vi "Conv1D.vi"() -> ()   [LabVIEW 2020]
doc: "This benchmark is designed to demonstrate execution performance improvement when executing FFT and IFFT operations on a GPU."
uses:
  956bade7-a26b-4376-82d1-4f43b9b25d0c.vi
  a45b64e6-426e-4566-b00d-58499d731ec9.vi
  2d4acfdf-3b2f-4360-8aac-546d4cc334b7.vi
  e3d6266a-341e-462f-8124-2d714a455819.vi
  <vilib>/Analysis/2dsp.llb/1D Convolution (DBL).vi
  <vilib>/Utility/High Resolution Relative Seconds.vi
  <vilib>/Ngene/CuLab - GPU Accelerated Toolkit/Toolkit/Low_Level/Tensor_Classes/T_Children/T1D/T1D_Children/T1D_SGL/Pull.vi
  <vilib>/Ngene/CuLab - GPU Accelerated Toolkit/Toolkit/API/Signal Processing/Signal Operation/Convolution/T1D/CU_Convolution_T1D_SGL.vi
  <vilib>/Ngene/CuLab - GPU Accelerated Toolkit/Toolkit/Low_Level/Tensor_Classes/T_Children/T1D/T1D_Children/T1D_SGL/Push.vi
  <vilib>/Ngene/CuLab - GPU Accelerated Toolkit/Toolkit/Low_Level/Tensor_Classes/T_Children/T1D/T1D_Children/T1D_SGL/Create_Push.vi
  <vilib>/Analysis/NI_AALBase.lvlib
  <vilib>/Ngene/CuLab - GPU Accelerated Toolkit/Toolkit/CuLab.lvlib
  <vilib>/Analysis/NI_AALPro.lvlib
  <vilib>/Ngene/CuLab - GPU Accelerated Toolkit/Toolkit/Low_Level/Tensor_Classes/T_Children/T1D/T1D_Children/T1D_SGL/T1D_SGL.lvclass
panel:
  out "CPU (sec)":dbl[](array[numeric])=[42.131092355985324, 35.429105230316075, 31.16246342351057, 25.767502048252396, 19.87054670676759, 14.576277208271852, 12.74999997084953, 7.518399561317554, 3.7424450318208833, 2.0503842820924176, 0.9362123659453822, 0.46770236324055325, 0.27725117698960117, 0.09920318843476397, 0.09302326738770976, 0.05329593103290103, 0.030920595781795512] format="%_3p"
  out "GPU (sec)":dbl[](array[numeric])=[42.131092355985324, 35.429105230316075, 31.16246342351057, 25.767502048252396, 19.87054670676759, 14.576277208271852, 12.74999997084953, 7.518399561317554, 3.7424450318208833, 2.0503842820924176, 0.9362123659453822, 0.46770236324055325, 0.27725117698960117, 0.09920318843476397, 0.09302326738770976, 0.05329593103290103, 0.030920595781795512] format="%_3p"
  out "Kernel Sizes":i32[](array[numeric])=[8389, 4195, 2098, 1049, 525, 263, 132, 66, 33, 17, 9, 5, 3, 3, 3, 3, 3] format="%#.7f"
  out "SpeedUp":dbl[](array[numeric])=[42.131092355985324, 35.429105230316075, 31.16246342351057, 25.767502048252396, 19.87054670676759, 14.576277208271852, 12.74999997084953, 7.518399561317554, 3.7424450318208833, 2.0503842820924176, 0.9362123659453822, 0.46770236324055325, 0.27725117698960117, 0.09920318843476397, 0.09302326738770976, 0.05329593103290103, 0.030920595781795512] format="%.2f"
  in  "Kernel Relative Size":sgl=0.001
  out "Iteration":i32=9
  out "FFT_Size":i32=128
  out "Status":string="Computing on CPU"
  out "GPU Model":string="NVIDIA GeForce GTX 1650 Ti"
  out "CPU Model":string="Intel(R) Core(TM) i7-10750H CPU @ 2.60GHz  "
  in  "No. of Repetitions":i32=10
  in  "Signal Size Stop (2^N)":i32=23
  in  "Signal Size Start (2^N)":i32=7
  out "Signal Sizes":i32[](array[numeric])=[8388608, 4194304, 2097152, 1048576, 524288, 262144, 131072, 65536, 32768, 16384, 8192, 4096, 2048, 1024, 512, 256, 128] format="%#.4f"
  out "Performance Improvement":cluster{i32[], dbl[]}(graph)={[8388608, 4194304, 2097152, 1048576, 524288, 262144, 131072, 65536, 32768, 16384, 8192, 4096, 2048, 1024, 512, 256, 128], [42.131092355985324, 35.429105230316075, 31.16246342351057, 25.767502048252396, 19.87054670676759, 14.576277208271852, 12.74999997084953, 7.518399561317554, 3.7424450318208833, 2.0503842820924176, 0.9362123659453822, 0.46770236324055325, 0.27725117698960117, 0.09920318843476397, 0.09302326738770976, 0.05329593103290103, 0.030920595781795512]}
  out "Execution Times":cluster{i32[], "FFT mean Exec Time":dbl[]}[](graph)=[{[8388608, 4194304, 2097152, 1048576, 524288, 262144, 131072, 65536, 32768, 16384, 8192, 4096, 2048, 1024, 512, 256, 128], "FFT mean Exec Time"=[0.8448884999997972, 0.3735822000016924, 0.16075780000028317, 0.06971139999950537, 0.02983959999983199, 0.012325700001383666, 0.005569199998717522, 0.00257430000056047, 0.0010898000000452157, 0.0004802000003110152, 0.00023630000214325264, 0.00011439999798312783, 5.8499997976468876e-05, 2.4900000425986946e-05, 1.3600001693703234e-05, 7.599999662488699e-06, 4.400000761961564e-06]}, {[8388608, 4194304, 2097152, 1048576, 524288, 262144, 131072, 65536, 32768, 16384, 8192, 4096, 2048, 1024, 512, 256, 128], "FFT mean Exec Time"=[0.020053800002642674, 0.01054449999719509, 0.005158699997991789, 0.002705399998376379, 0.0015017000005173031, 0.0008455999995931052, 0.00043680000089807436, 0.0003423999987717252, 0.00029120000181137584, 0.0002342000007047318, 0.00025240000104531646, 0.0002445999998599291, 0.00021099999867146835, 0.00025100000129896216, 0.00014620000001741573, 0.00014259999807109125, 0.00014229999942472205]}]
  # "Overview: Benchmarks performance of a GPU vs CPU in 1D Convolution task.\nRequirements: PC with Nvidia GPU, with latest version of GPU driver and CuLab Toolkit installed.\nInstructions:\n1. Run the VI with the current benchmarking parameters.\n2. Wait for the completion of the execution. \nNote: It might take some time to perform the computations.\n3. Observe the timing and speedup results on the graphs."
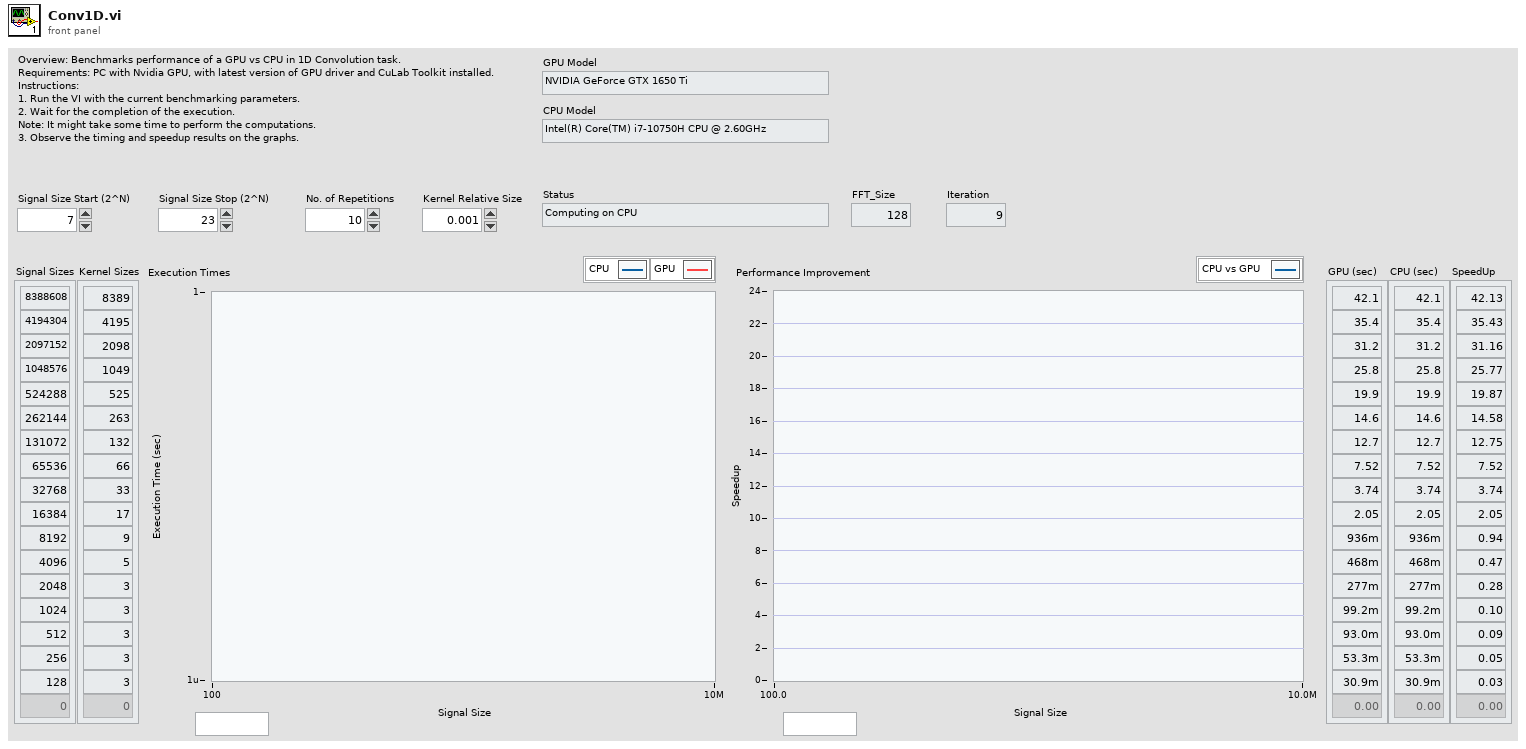
[diagram p1: front panel]
types:
  T1 = typedef "CuLab.lvlib/Properties.ctl" = cluster{"Index":i32, "Name":string}
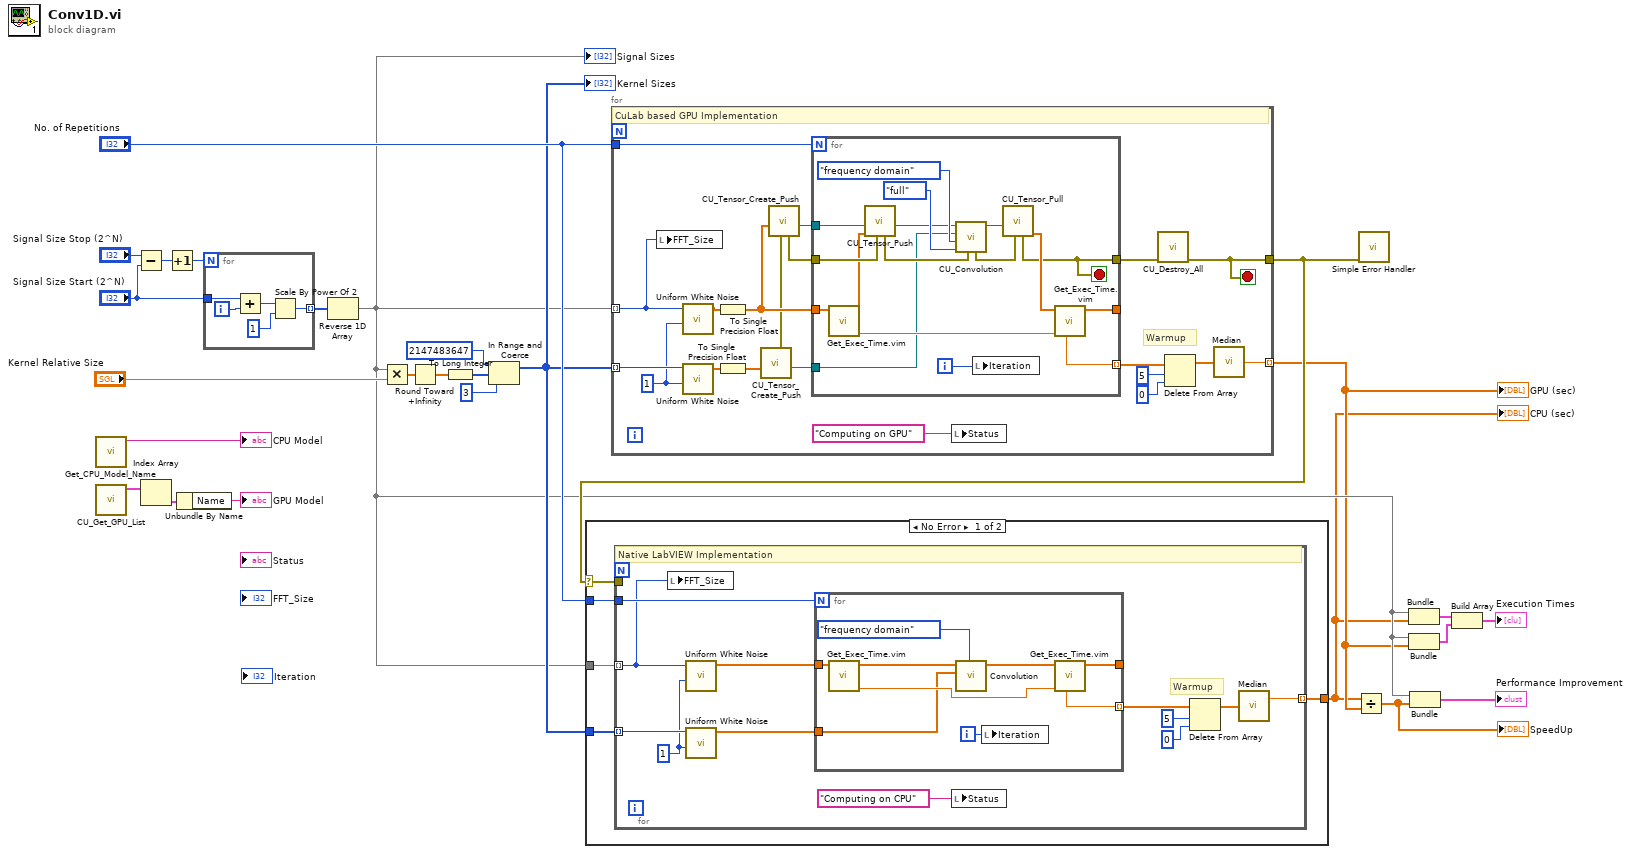
[diagram p0: block diagram]
diagram:
  n1 = call "Get_CPU_Model_Name.vi"() -> ("CPU Model"=→"CPU Model":string)  [unwired: 11 in]
  n2 = call <vilib>:"CU_Get_GPU_List.vi"() -> ("Devices"=w6:T1[])  [unwired: 10 in, 1 out]
  n3 = Subtract(x="Signal Size Stop (2^N)", y="Signal Size Start (2^N)") -> (x-y=w21:i32)
  n4 = Index Array(array=w6) -> (element=w5:T1)  [unwired: 1 in]
  n5 = Increment(x=w21) -> (x+1=w20:i32)
  n6 = Unbundle By Name(w5) -> ("Name"=→"GPU Model":string)
  n7 = for {
    N: w20 -> [_]
    tunnel: "Signal Size Start (2^N)" -> [w31]
    tunnel: [w27] -> w8 mode=indexing
    i -> [w30]
    n8 = Add(x=w31, y=w30) -> (x+y=w29:i32)
    n9 = Scale By Power Of 2(n=w29, x=1) -> (x*2^n=w27:i32)
  }
  n10 = Reverse 1D Array(array=w8) -> (reversed array=w3:i32[])
  "Signal Sizes" <- w3
  n11 = Multiply(x=w3, y="Kernel Relative Size") -> (x*y=w14:sgl[])
  n12 = Round Toward +Infinity(x=w14) -> (ceil(x): smallest int >= x=w13:sgl[])
  n13 = To Long Integer(number=w13) -> (32bit integer=w11:i32[])
  n14 = In Range and Coerce(upper limit=2147483647 ("lower limit"), x=w11, lower limit=3) -> (coerced(x)=w12:i32[])  [unwired: 1 out]
  "Kernel Sizes" <- w12
  n15 = for {
    tunnel: [w41] -> w17
    tunnel: [w49] -> w2 mode=indexing
    tunnel: w3 -> [w39] mode=indexing
    tunnel: "No. of Repetitions" -> [w45]
    tunnel: w12 -> [w33] mode=indexing
    stop <- w41 stop-if-true
    w32 = 1 ("seed")
    # "Warmup"
    # "CuLab based GPU Implementation"
    n16 = local write "FFT_Size"(w39) -> ()
    n17 = call <vilib>:"Uniform White Noise.vi"("seed"=w32, "samples"=w39) -> ("uniform white noise"=w42:dbl[])  [unwired: 8 in, 1 out]
    n18 = call <vilib>:"Uniform White Noise.vi"("seed"=w32, "samples"=w33) -> ("uniform white noise"=w38:dbl[])  [unwired: 8 in, 1 out]
    n19 = To Single Precision Float(number=w42) -> (single precision float=w43:sgl[])
    n20 = To Single Precision Float(number=w38) -> (single precision float=w37:sgl[])
    n21 = call-poly <vilib>:"CU_Tensor_Create_Push.vi"("CPU_Data_1D_SGL"=w37) -> ("T1D_SGL out"=w36:refnum<class "T1D_SGL.lvclass">, "error out"=w35:errorcluster)  [unwired: 9 in]
    n22 = call-poly <vilib>:"CU_Tensor_Create_Push.vi"("error in (no error)"=w35, "CPU_Data_1D_SGL"=w43) -> ("T1D_SGL out"=w51:refnum<class "T1D_SGL.lvclass">, "error out"=w50:errorcluster)  [unwired: 8 in]
    n23 = for {
      N: w45 -> [_]
      tunnel: w51 -> [w65]
      tunnel: w50 -> [w57]
      tunnel: [w52] -> w44
      tunnel: [w66] -> w34 mode=indexing
      tunnel: w43 -> [w56]
      tunnel: w36 -> [w58]
      tunnel: [w54] -> _
      i -> [w62]
      stop <- w52 stop-if-true
      n24 = call "Get_Exec_Time.vim"("error in (no error)"=w56) -> ("T(n)"=w67:dbl, "error out"=w55:sgl[])  [unwired: 6 in, 1 out]
      n25 = call-poly <vilib>:"CU_Tensor_Push.vi"("error in (no error)"=w57, "CPU_Data_1D_SGL"=w55, "T1D_SGL in"=w65) -> ("T1D_SGL out"=w59:refnum<class "T1D_SGL.lvclass">, "error out"=w68:errorcluster)  [unwired: 7 in]
      n26 = call-poly <vilib>:"CU_Convolution.vi"("error in"=w68, "output size"=enum32{"full", "size X", "compact"}."full", "algorithm"=enum32{"direct", "frequency domain"}."frequency domain", "Y"=w58, "X"=w59) -> ("X * Y"=w64:refnum<class "T1D_SGL.lvclass">, "error out"=w63:errorcluster)  [unwired: 5 in]
      n27 = local write "Iteration"(w62) -> ()
      n28 = call-poly <vilib>:"CU_Tensor_Pull.vi"("error in (no error)"=w63, "T1D_SGL in"=w64) -> ("Dest out"=w53:sgl[], "error out"=w52:errorcluster)  [unwired: 7 in, 1 out]
      n29 = call "Get_Exec_Time.vim"("T(n-1)"=w67, "error in (no error)"=w53) -> ("error out"=w54:sgl[], "dT"=w66:dbl)  [unwired: 5 in, 1 out]
    }
    n30 = local write "Status"("Computing on GPU" ("Info")) -> ()
    n31 = call <vilib>:"CU_Destroy_All.vi"("error in"=w44) -> ("error out"=w41:errorcluster)  [unwired: 10 in]
    n32 = Delete From Array(array=w34, length=5, index=0) -> (array with subset deleted=w48:dbl[])  [unwired: 1 out]
    n33 = call <vilib>:"Median.vi"("X"=w48) -> ("median"=w49:dbl)  [unwired: 1 out]
  }
  "GPU (sec)" <- w2
  n34 = case shown="No Error" w17 {
    selector: w17 -> [w70 _]
    tunnel: [w73 _] -> w1
    tunnel: "No. of Repetitions" -> [w72 _]
    tunnel: w3 -> [w71 _]
    tunnel: w12 -> [w69 _]
    frame No Error {
      n35 = for {
        tunnel: [w81] -> w73 mode=indexing
        tunnel: w71 -> [w77] mode=indexing
        tunnel: w72 -> [w80]
        tunnel: w70 -> [_]
        tunnel: w69 -> [w76] mode=indexing
        w74 = 1 ("seed")
        # "Warmup"
        # "Native LabVIEW Implementation"
        n36 = local write "FFT_Size"(w77) -> ()
        n37 = call <vilib>:"Uniform White Noise.vi"("seed"=w74, "samples"=w77) -> ("uniform white noise"=w79:dbl[])  [unwired: 8 in, 1 out]
        n38 = call <vilib>:"Uniform White Noise.vi"("seed"=w74, "samples"=w76) -> ("uniform white noise"=w75:dbl[])  [unwired: 8 in, 1 out]
        n39 = for {
          N: w80 -> [_]
          tunnel: w79 -> [w94]
          tunnel: [w93] -> _
          tunnel: [w91] -> w85 mode=indexing
          tunnel: w75 -> [w86]
          i -> [w90]
          n40 = call "Get_Exec_Time.vim"("error in (no error)"=w94) -> ("T(n)"=w92:dbl, "error out"=w89:dbl[])  [unwired: 6 in, 1 out]
          n41 = call-poly <vilib>:"Convolution.vi"("algorithm"=enum32{"direct", "frequency domain"}."frequency domain", "Y"=w86, "X"=w89) -> ("X * Y"=w88:dbl[])  [unwired: 7 in, 1 out]
          n42 = local write "Iteration"(w90) -> ()
          n43 = call "Get_Exec_Time.vim"("T(n-1)"=w92, "error in (no error)"=w88) -> ("error out"=w93:dbl[], "dT"=w91:dbl)  [unwired: 5 in, 1 out]
        }
        n44 = local write "Status"("Computing on CPU" ("Info")) -> ()
        n45 = Delete From Array(array=w85, length=5, index=0) -> (array with subset deleted=w82:dbl[])  [unwired: 1 out]
        n46 = call <vilib>:"Median.vi"("X"=w82) -> ("median"=w81:dbl)  [unwired: 1 out]
      }
    }
    frame Error {
    }
  }
  "CPU (sec)" <- w1
  n47 = Divide(x=w1, y=w2) -> (x/y=w15:dbl[])
  "SpeedUp" <- w15
  n48 = call <vilib>:"Simple Error Handler.vi"("error in (no error)"=w17) -> ()  [unwired: 4 in, 5 out]
  n49 = Bundle(w3, w1) -> (w26:cluster{i32[], dbl[]})  [unwired: 1 in]
  n50 = Bundle(w3, w2) -> (w25:cluster{i32[], dbl[]})  [unwired: 1 in]
  n51 = Bundle(w3, w15) -> (→"Performance Improvement":cluster{i32[], dbl[]})  [unwired: 1 in]
  n52 = Build Array(w26, w25) -> (→"Execution Times":cluster{i32[], dbl[]}[])
